vi "MOSES.vi"(7 "Scan List (empty)":string="101:132,201:222", 8 "error in (no error)":errorcluster, 9 "Range (5:Auto)":T3(ring)=enum."Auto", 10 "Resolution (5:Default)":T2(ring)=enum."Default", 11 "VISA resource name":refnum<visa-resource-name>="GPIB0::9::INSTR") -> (0 "error out":errorcluster, 2 "Output Array":dbl[](array[numeric]) format="%.2f", 3 "VISA resource name out":refnum<visa-resource-name>)   [LabVIEW 2013]
doc: "This VI allows you to take simple voltage measurements from the instrument."
uses:
  Instance           7 13Saved   MOSES .vi
  Instance           2 13Saved   MOSES .vi
  Instance          24 13Saved   MOSES .vi
  Instance          83 13Saved   MOSES .vi
  Instance          81 13Saved   MOSES .vi
  Instance          79 13Saved   MOSES .vi
  Instance          77 13Saved   MOSES .vi
  Instance          75 13Saved   MOSES .vi
  Instance          71 13Saved   MOSES .vi
  Instance          69 13Saved   MOSES .vi
  Instance          67 13Saved   MOSES .vi
  Instance          65 13Saved   MOSES .vi
  Instance          63 13Saved   MOSES .vi
  Instance          61 13Saved   MOSES .vi
  Instance          59 13Saved   MOSES .vi
  Instance          57 13Saved   MOSES .vi
  Instance          55 13Saved   MOSES .vi
  Instance          53 13Saved   MOSES .vi
  Instance          51 13Saved   MOSES .vi
  Instance          49 13Saved   MOSES .vi
  Instance          47 13Saved   MOSES .vi
  Instance          42 13Saved   MOSES .vi
  Instance          40 13Saved   MOSES .vi
  Instance          38 13Saved   MOSES .vi
  Instance          36 13Saved   MOSES .vi
  Instance          34 13Saved   MOSES .vi
  Instance          32 13Saved   MOSES .vi
  Instance          30 13Saved   MOSES .vi
  Instance          28 13Saved   MOSES .vi
  Instance          26 13Saved   MOSES .vi
  Instance          22 13Saved   MOSES .vi
  Instance          20 13Saved   MOSES .vi
  Instance          18 13Saved   MOSES .vi
  Instance          16 13Saved   MOSES .vi
  Instance          14 13Saved   MOSES .vi
  Instance          12 13Saved   MOSES .vi
  Instance          10 13Saved   MOSES .vi
  Instance           8 13Saved   MOSES .vi
  <vilib>/express/express shared/transition.llb/Dynamic To Waveform Array.vi
  <vilib>/express/express shared/transition.llb/Waveform Array To Dynamic.vi
  <vilib>/express/express arith-compare/Formula/Block/exnFormulaBlock how many pts in the wave.vi
  <vilib>/express/express shared/ex_Modify Signal Name.vi
  <vilib>/express/express arith-compare/Formula/XNode/ExpressFormulaBlockNode.xnode
panel:
  in  "?":bool
  in  "?":T1(tab)
  out "TEC L -y":dbl
  out "Battery":dbl
  out "Boolean 10":bool
  out "Boolean 11":bool
  out "Boolean 12":bool
  out "Mains from IS":dbl
  out "Boolean 13":bool
  out "Boolean 14":bool
  out "Boolean 15":bool
  out "12d+, MTR2812D Out":dbl
  out "Boolean 16":bool
  out "Boolean 17":bool
  out "5s, MGA2805S Out":dbl
  out "Boolean 26":bool
  out "Boolean 27":bool
  out "IS Out":dbl
  out "Boolean 20":bool
  out "Boolean 21":bool
  out "Boolean 22":bool
  out "12d+ MTR2812D Out":dbl
  out "Boolean 23":bool
  out "Boolean 24":bool
  out "Boolean 25":bool
  out "5s MGA2805S Out":dbl
  out "Boolean 29":bool
  out "Boolean 30":bool
  out "Boolean 31":bool
  out "Power Supply Filter Input":dbl
  out "Boolean 67":bool
  out "Boolean 68":bool
  out "Boolean 90":bool
  out "Boolean 7":bool
  out "Boolean 8":bool
  out "TEC L +y":dbl
  out "Boolean 6":bool
  out "Boolean 5":bool
  out "TEC L 0y":dbl
  out "Boolean 9":bool
  out "Boolean 18":bool
  out "TEC R +y":dbl
  out "Boolean 19":bool
  out "Boolean 45":bool
  out "TEC R -y":dbl
  out "Boolean 46":bool
  out "Boolean 75":bool
  out "TEC R 0y":dbl
  out "Boolean 76":bool
  out "Boolean 89":bool
  out "Thermal 5V power":dbl
  out "Shutter 28V power":dbl
  out "H-alpha filter":dbl
  out "H-alpha camera":dbl
  out "ROE power supply input":dbl
  out "Premod filter positive 12V input":dbl
  out "Premod filter 5V input":dbl
  out "Shutter 28V power":dbl
  out "H-alpha filter":dbl
  out "ROE power supply input":dbl
  out "Boolean 41":bool
  out "Boolean 42":bool
  out "Res +y":dbl
  out "Res -y":dbl
  out "Res Back":dbl
  out "Boolean 43":bool
  out "Boolean 44":bool
  out "Boolean 47":bool
  out "Boolean 48":bool
  out "Boolean 49":bool
  out "Boolean 50":bool
  out "CF +y":dbl
  out "CF -y":dbl
  out "CF 0y":dbl
  out "Boolean 51":bool
  out "Boolean 52":bool
  out "Boolean 53":bool
  out "Boolean 54":bool
  out "BP +y":dbl
  out "BP -y":dbl
  out "BP 0y":dbl
  out "Boolean 55":bool
  out "Boolean 56":bool
  out "Boolean 57":bool
  out "Boolean 58":bool
  out "Boolean 59":bool
  out "Boolean 60":bool
  out "Boolean 40":bool
  out "PCU Res":dbl
  out "Boolean 83":bool
  out "Boolean 84":bool
  out "ICU":dbl
  out "Boolean 85":bool
  out "Boolean 86":bool
  out "PCU Box":dbl
  out "Boolean 87":bool
  out "Boolean 88":bool
  out "Boolean 32":bool
  out "Boolean 33":bool
  out "Boolean 34":bool
  out "TEC +y":dbl
  out "TEC -y":dbl
  out "TEC 0y":dbl
  out "Boolean 35":bool
  out "Boolean 36":bool
  out "Boolean 37":bool
  out "Boolean 38":bool
  out "Boolean 39":bool
  out "Comp Res":dbl
  out "Boolean 61":bool
  out "Boolean 62":bool
  out "Vortec x86 CPU":dbl
  out "Boolean 63":bool
  out "Boolean 64":bool
  out "Mainboard":dbl
  out "Boolean 65":bool
  out "Boolean 66":bool
  out "Virtex 5 FPGA":dbl
  out "Boolean 69":bool
  out "Boolean 70":bool
  out "RPA":dbl
  out "Boolean 71":bool
  out "Boolean 72":bool
  out "TC Res.":dbl
  out "Boolean 73":bool
  out "Boolean 74":bool
  out "T CONT b -y":dbl
  out "Boolean 77":bool
  out "Boolean 78":bool
  out "12S":dbl
  out "Boolean 79":bool
  out "Boolean 80":bool
  out "12D":dbl
  out "Boolean 81":bool
  out "Boolean 82":bool
  out "0 Order TECs":dbl[][](graph)
  out "-1 Order TECs":dbl[][](graph)
  out "+1 Order TECs":dbl[][](graph)
  out "I5s":dbl[](graph)
  out "I12d+":dbl[](graph)
  out "Iout":dbl[](graph)
  out "Power Supply Filter Input":dbl[](graph)
  out "TEC Currents":dbl[][](graph)
  out "Back Plates":dbl[][](graph)
  out "Cold Fingers":dbl[][](graph)
  out "CONT":dbl[][](graph)
  out "PCU":dbl[][](graph)
  out "COMP":dbl[][](graph)
  out "Reservoir":dbl[][](graph)
  out "ROE":dbl[](graph)
  out "PSU":dbl[](graph)
  in  "C":dbl
  in  "B":dbl
  in  "A":dbl
  in  "stop 2":bool
  # "System"
  # "System"
  # "Voltage"
  # "Current"
  # "C"
  # "V"
  # "A"
  # "Temperatures of \n+1 Order CCD\nThermal Reservoir, Cold Finger, and Back Plate"
  # "C"
  # "A"
  # "V"
  # "C"
  # "A"
  # "V"
  # "Temperatures of \n0 Order CCD\nCold Finger and Back Plate"
  # "C"
  # "V"
  # "mA"
  # "C"
  # "Thermo Electric Coolers (TEC)"
  # "CCD"
  # "Voltage on L or R side of TEC"
  # "Current"
  # "C"
  # "Temperatures of \n-1 Order CCD\nThermal Reservoir, Cold Finger, and Back Plate"
  # "V"
  # "C"
  # "+1 Order"
  # "A"
  # "V"
  # "C"
  # "Temperature of\nBack of Thermal Reservoir"
  # "C"
  # "V"
  # "0 Order"
  # "A"
  # "Computer"
  # "V"
  # "C"
  # "C"
  # "C"
  # "V"
  # "-1 Order"
  # "A"
  # "C"
  # "C"
  # "C"
  # "V"
  # "Sub-Systems"
  # "C"
  # "C"
  # "Current"
  # "Voltage"
  # "C"
  # "C"
  # "mA"
  # "V"
  # "C"
  # "C"
  # "V"
  # "mA"
  # "V"
  # "A"
  # "V"
  # "A"
  # "V"
  # "A"
  # "Please add graphs and values that you would like to see in the text box below."
  # "Flight Screen:\n-TECs\n-\n-"
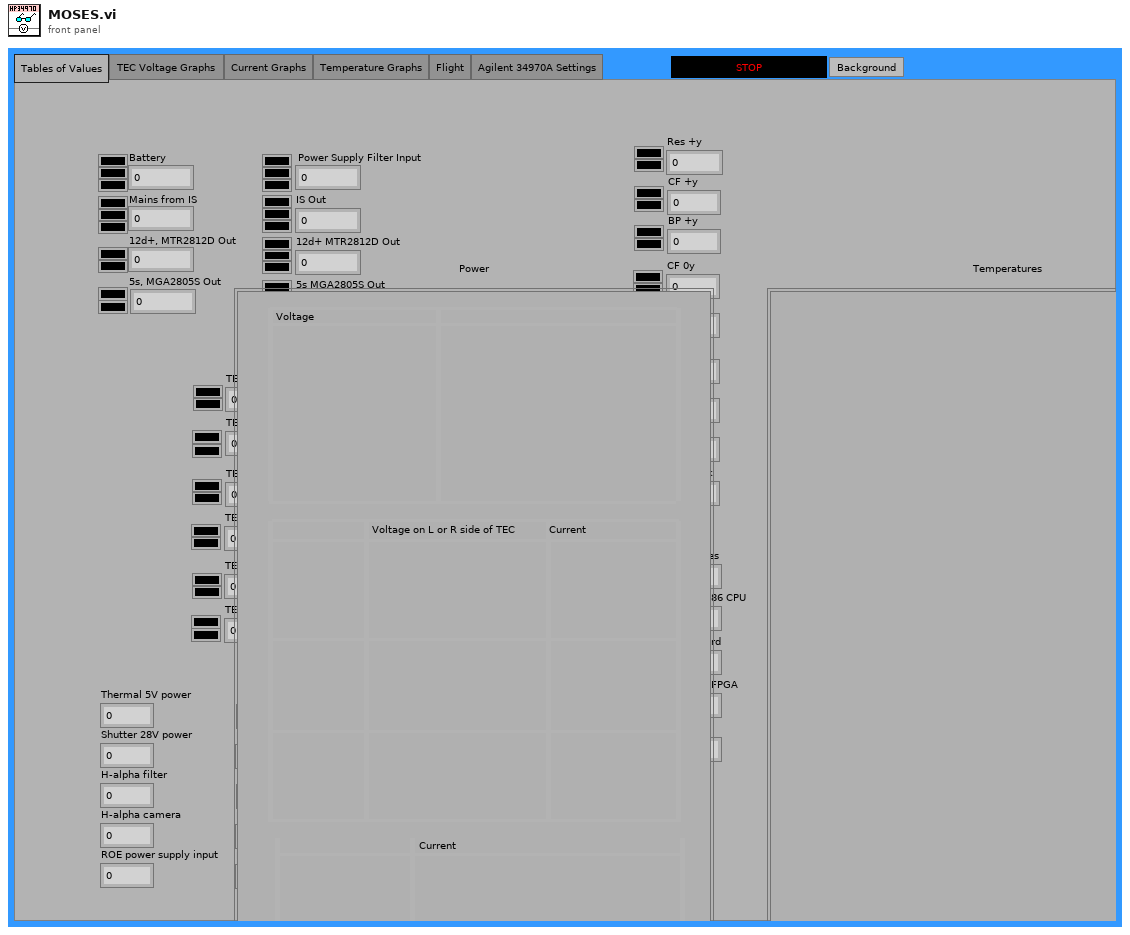
[diagram p1: front panel]
types:
  T1 = enum32{"Tables of Values", "TEC Voltage Graphs ", "Current Graphs", "Temperature Graphs", "Flight", "Agilent 34970A Settings"}
  T2 = enum16{"4 1/2", "5 1/2", "6 1/2", "Least", "Highest", "Default"}
  T3 = enum16{"100 mV", "1 V", "10 V", "100 V", "300 V", "Auto", "Minimum", "Maximum"}
  T4 = cluster{"Output Number Array[0]":dbl, "Output Number Array[1]":dbl, "Output Number Array[2]":dbl, "Output Number Array[3]":dbl, "Output Number Array[4]":dbl, "Output Number Array[5]":dbl, "Output Number Array[6]":dbl, "Output Number Array[7]":dbl, "Output Number Array[8]":dbl, "Output Number Array[9]":dbl, "Output Number Array[10]":dbl, "Output Number Array[11]":dbl, "Output Number Array[12]":dbl, "Output Number Array[13]":dbl, "Output Number Array[14]":dbl, "Output Number Array[15]":dbl, "Output Number Array[16]":dbl, "Output Number Array[17]":dbl, "Output Number Array[18]":dbl, "Output Number Array[19]":dbl, "Output Number Array[20]":dbl, "Output Number Array[21]":dbl, "Output Number Array[22]":dbl, "Output Number Array[23]":dbl, "Output Number Array[24]":dbl, "Output Number Array[25]":dbl, "Output Number Array[26]":dbl, "Output Number Array[27]":dbl, "Output Number Array[28]":dbl, "Output Number Array[29]":dbl, "Output Number Array[30]":dbl, "Output Number Array[31]":dbl, "Output Number Array[32]":dbl, "Output Number Array[33]":dbl, "Output Number Array[34]":dbl, "Output Number Array[35]":dbl, "Output Number Array[36]":dbl, "Output Number Array[37]":dbl, "Output Number Array[38]":dbl, "Output Number Array[39]":dbl, "Output Number Array[40]":dbl, "Output Number Array[41]":dbl, "Output Number Array[42]":dbl, "Output Number Array[43]":dbl, "Output Number Array[44]":dbl, "Output Number Array[45]":dbl, "Output Number Array[46]":dbl, "Output Number Array[47]":dbl, "Output Number Array[48]":dbl, "Output Number Array[49]":dbl, "Output Number Array[50]":dbl, "Output Number Array[51]":dbl, "Output Number Array[52]":dbl, "Output Number Array[53]":dbl, "Output Number Array[54]":dbl, "Output Number Array[55]":dbl, "Output Number Array[56]":dbl, "Output Number Array[57]":dbl, "Output Number Array[58]":dbl, "Output Number Array[59]":dbl, "Output Number Array[60]":dbl, "Output Number Array[61]":dbl, "Output Number Array[62]":dbl, "Output Number Array[63]":dbl, "Output Number Array[64]":dbl, "Output Number Array[65]":dbl, "Output Number Array[66]":dbl, "Output Number Array[67]":dbl, "Output Number Array[68]":dbl, "Output Number Array[69]":dbl}
  T5 = cluster{"V5s, MGA2805S output voltage":dbl, "T5V, Thermal 5V power voltage":dbl, "S28V, Shutter 28V power voltage":dbl, "HAFV, H-alpha filter voltage":dbl, "HACV, H-alpha camera voltage":dbl, "If_in, Power supply filter input current":dbl, "Ipf12+, Premod filter positive 12V input current":dbl, "I_pf5, Premod filter 5V input current":dbl, "S28I, Shutter 28V power current":dbl, "HAFI, H-alpha filter current":dbl, "ROE_PSV, ROE power supply input voltage":dbl, "ROE_PSI, ROE power supply input current":dbl, "T_ROE, ROE Temp.":dbl, "T_PSU, PSU Temp.":dbl}
diagram:
  # "This goes to MOSES background."
  n1 = while {
    shift-right: [w645] -> _
    shift-left: _ -> [w646]
    shift-right: [w1] -> _
    shift-left: _ -> [w637]
    shift-right: [w635] -> _
    shift-left: _ -> [w636]
    shift-right: [w2] -> _
    shift-left: _ -> [w620]
    shift-right: [w3] -> _
    shift-left: _ -> [w618]
    shift-right: [w4] -> _
    shift-left: _ -> [w597]
    shift-right: [w5] -> _
    shift-left: _ -> [w593]
    shift-right: [w6] -> _
    shift-left: _ -> [w182]
    shift-right: [w7] -> _
    shift-left: _ -> [w580]
    shift-right: [w8] -> _
    shift-left: _ -> [w563]
    shift-right: [w9] -> _
    shift-left: _ -> [w532]
    shift-right: [w10] -> _
    shift-left: _ -> [w511]
    shift-right: [w505] -> _
    shift-left: _ -> [w506]
    shift-right: [w463] -> _
    shift-left: _ -> [w462]
    shift-right: [w461] -> _
    shift-left: _ -> [w460]
    shift-right: [w457] -> _
    shift-left: _ -> [w458]
    shift-right: [w456] -> _
    shift-left: _ -> [w455]
    shift-right: [w454] -> _
    shift-left: _ -> [w453]
    shift-right: [w452] -> _
    shift-left: _ -> [w451]
    shift-right: [w450] -> _
    shift-left: _ -> [w449]
    shift-right: [w448] -> _
    shift-left: _ -> [w183]
    shift-right: [w447] -> _
    shift-left: _ -> [w446]
    shift-right: [w445] -> _
    shift-left: _ -> [w444]
    shift-right: [w443] -> _
    shift-left: _ -> [w442]
    shift-right: [w63] -> _
    shift-left: _ -> [w176]
    shift-right: [w434] -> _
    shift-left: _ -> [w433]
    shift-right: [w89] -> _
    shift-left: _ -> [w435]
    shift-right: [w432] -> _
    shift-left: _ -> [w431]
    shift-right: [w430] -> _
    shift-left: _ -> [w429]
    shift-right: [w11] -> _
    shift-left: _ -> [w368]
    shift-right: [w366] -> _
    shift-left: _ -> [w367]
    shift-right: [w365] -> _
    shift-left: _ -> [w364]
    shift-right: [w363] -> _
    shift-left: _ -> [w362]
    shift-right: [w360] -> _
    shift-left: _ -> [w361]
    shift-right: [w356] -> _
    shift-left: _ -> [w357]
    shift-right: [w359] -> _
    shift-left: _ -> [w358]
    shift-right: [w12] -> _
    shift-left: _ -> [w316]
    shift-right: [w314] -> _
    shift-left: _ -> [w313]
    shift-right: [w312] -> _
    shift-left: _ -> [w311]
    shift-right: [w309] -> _
    shift-left: _ -> [w310]
    shift-right: [w308] -> _
    shift-left: _ -> [w307]
    shift-right: [w273] -> _
    shift-left: _ -> [w274]
    shift-right: [w272] -> _
    shift-left: _ -> [w271]
    shift-right: [w269] -> _
    shift-left: _ -> [w270]
    shift-right: [w13] -> _
    shift-left: _ -> [w275]
    stop <- "stop 2" stop-if-true
    w75 = 0.05 ("y")
    w76 = 4.0 ("y")
    w81 = 2.5 ("y")
    w119 = 2.5 ("y")
    w123 = 2.5 ("y")
    w127 = 2.5 ("y")
    w130 = 2.5 ("y")
    (unwired) 37482.0 ("double precision float")
    (unwired) 9360000.0 ("double precision float")
    (unwired) 9.3e-08 ("double precision float")
    (unwired) 0.000236053 ("double precision float")
    (unwired) 9.3e-08 ("double precision float")
    (unwired) 0.000236053 ("double precision float")
    (unwired) 0.001285847 ("double precision float")
    (unwired) 0.001285847 ("double precision float")
    w69 = 150.0 ("y")
    w73 = 300.0 ("y")
    w104 = 2.5 ("y")
    w22 = 0.03 ("y")
    w109 = 3.0 ("y")
    w29 = 0.01 ("y")
    w639 = 2.5 ("y")
    w641 = 2.5 ("y")
    # "File saves to data.txt on the desktop."
    # "These four need real equations and alarm limits."
    # "For highest resolution\nmeasurements, \nchange VISA timeout"
    n2 = Append True/False String(1:FALSE ("selector"), 2:"DC? ", 3:"AC? ", 4:"MEAS:VOLT:") -> (0:w653:string)
    n3 = Pick Line(string ("")=w653, multi-line string=".1,\n1,\n10,\n100,\n300,\nAUTO\nMIN,\nMAX,", line index="Range (5:Auto)") -> (output string=w650:string)
    n4 = case shown="Default" "Range (5:Auto)" {
      selector: "Range (5:Auto)" -> [_ w1550]
      tunnel: [w1544 w1547] -> w649
      tunnel: w650 -> [w1544 w1546]
      tunnel: "Resolution (5:Default)" -> [_ w1548]
      frame "Auto" {
        # "Autorange"
      }
      frame Default {
        # "Not Autorange"
        n5 = Index Array(array=dbl[] [0.1, 1.0, 10.0, 100.0, 300.0, 0.0, 0.1, 300.0], index=w1550) -> (element=w1545:dbl)
        n6 = case shown="Default" w1548 {
          selector: w1548 -> [w1557 _ _ _]
          tunnel: [w1551 w1561 w1564 w1565] -> w1547
          tunnel: w1546 -> [w1554 w1560 w1562 w1566]
          tunnel: w1545 -> [w1556 _ _ _]
          frame Default {
            # "4.5, 5.5, or 6.5 Digits *"
            n7 = Index Array(array=dbl[] [0.0001, 3e-06, 1e-06], index=w1557) -> (element=w1555:dbl)
            n8 = Multiply(x=w1555, y=w1556) -> (x*y=w1553:dbl)
            n9 = Format Into String(format string="%.; %e", initial string=w1554, w1553) -> (resulting string=w1551:string)  [unwired: 1 in, 1 out]
          }
          frame "Least" {
            # "Least resolution"
            n10 = Concatenate Strings(w1560, " MAX" ("string")) -> (w1561:string)
          }
          frame "Highest" {
            # "Highest range"
            n11 = Concatenate Strings(w1562, " MIN" ("string")) -> (w1564:string)
          }
          frame "Default" {
            # "Default range"
            n12 = Concatenate Strings(w1566, " DEF" ("string")) -> (w1565:string)
          }
        }
      }
    }
    n13 = call "Convert to Dynamic Data3"() -> ("Dynamic Data Type"=w577:dynamicdata)  [unwired: 4 in]
    n14 = xnode "Voltage - Resistance"("V1"=5000, "28V"=w577, "R1"=28) -> ("Result"=w572:dynamicdata)  [unwired: 1 in, 1 out]
    n15 = Concatenate Strings(w649, ", (@", "Scan List (empty)", ")") -> (w660:string)
    n16 = VISA Write(VISA resource name="VISA resource name", write buffer=w660, error in (no error)="error in (no error)") -> (VISA resource name out=w669:refnum<visa-resource-name>, error out=w668:errorcluster)  [unwired: 1 out]
    n17 = xnode "Steinhart-Hart"("X1"=5000, "X2"=5000, "X3"=5000, "X4"=w572) -> ("Result"=w578:dynamicdata)  [unwired: 1 in, 1 out]
    n18 = property class="Instr"(reference=w669, error in=w668, "General Settings:Timeout Value"=u32 320000 ("Tmo Value")) -> (reference out=w666:refnum<visa-resource-name>, error out=w667:errorcluster)
    n19 = call "Convert from Dynamic Data9"("Dynamic Data Type"=w578) -> ()  [unwired: 3 in, 1 out]
    n20 = Get Date/Time String(want seconds? (F)=TRUE) -> (time string=w648:string)  [unwired: 2 in, 1 out]
    n21 = VISA Read(VISA resource name=w666, byte count=u32 4088 ("byte count (0)"), error in (no error)=w667) -> (VISA resource name out=→"VISA resource name out":refnum<visa-resource-name>, read buffer=w661:string, error out=→"error out":errorcluster)  [unwired: 1 out]
    n22 = call <instrlib>:"HP34970A List to Array.vi"("List (empty)"=w661) -> ("Output Number Array"=w181:dbl[])  [unwired: 5 in, 1 out]
    "Output Array" <- w181
    n23 = call "sub_vi.vi"("Array"=w181) -> ("Dynamic Data Type"=w643:dynamicdata)  [unwired: 3 in]
    n24 = call "Write LabVIEW Measurement File2"("Comment"=w648, "Signals"=w643) -> ()  [unwired: 7 in, 3 out]
    n25 = Array To Cluster(array=w181) -> (cluster=w638:T4)
    n26 = Build Array (concatenate)(w646, w181) -> (w645:dbl[][])
    n27 = Unbundle(w638) -> ("Output Number Array[0]"=w134:dbl, "Output Number Array[1]"=w20:dbl, "Output Number Array[2]"=w132:dbl, "Output Number Array[3]"=w126:dbl, "Output Number Array[4]"=w122:dbl, "Output Number Array[5]"=w118:dbl, "Output Number Array[8]"=w140:dbl, "Output Number Array[9]"=w143:dbl, "Output Number Array[10]"=w146:dbl, "Output Number Array[11]"=w98:dbl, "Output Number Array[16]"=w175:dbl, "Output Number Array[17]"=w88:dbl, "Output Number Array[18]"=w174:dbl, "Output Number Array[19]"=w173:dbl, "Output Number Array[22]"=w172:dbl, "Output Number Array[23]"=w171:dbl, "Output Number Array[24]"=w170:dbl, "Output Number Array[29]"=w169:dbl, "Output Number Array[30]"=w168:dbl, "Output Number Array[32]"=w167:dbl, "Output Number Array[33]"=w166:dbl, "Output Number Array[34]"=w165:dbl, "Output Number Array[35]"=w164:dbl, "Output Number Array[36]"=w163:dbl, "Output Number Array[37]"=w162:dbl, "Output Number Array[38]"=w161:dbl, "Output Number Array[39]"=w160:dbl, "Output Number Array[40]"=w159:dbl, "Output Number Array[41]"=w158:dbl, "Output Number Array[42]"=w157:dbl, "Output Number Array[43]"=w156:dbl, "Output Number Array[44]"=w155:dbl, "Output Number Array[45]"=w154:dbl, "Output Number Array[46]"=w147:dbl, "Output Number Array[49]"=w151:dbl, "Output Number Array[50]"=w152:dbl, "Output Number Array[51]"=w150:dbl, "Output Number Array[52]"=w148:dbl, "Output Number Array[53]"=w149:dbl)  [unwired: 31 out]
    "TEC L +y" <- w134
    "TEC L 0y" <- w132
    "TEC R +y" <- w126
    "TEC R -y" <- w122
    "TEC R 0y" <- w118
    "TEC L -y" <- w20
    n28 = xnode "Votage - Current"("X1"=w172) -> ("Result"=w583:dbl)  [unwired: 1 in, 1 out]
    n29 = xnode "V -> T"("a"=0.001285847 ("double precision float"), "b"=0.000236053 ("double precision float"), "c"=9.3e-08 ("double precision float"), "R"=9360000.0 ("double precision float"), "v0"=w169) -> ("Result"=w566:dbl)  [unwired: 1 in, 1 out]
    n30 = xnode "V -> T"("a"=0.001285847 ("double precision float"), "b"=0.000236053 ("double precision float"), "c"=9.3e-08 ("double precision float"), "R"=9360000.0 ("double precision float"), "v0"=w167) -> ("Result"=w551:dbl)  [unwired: 1 in, 1 out]
    n31 = xnode "V -> T"("a"=0.001285847 ("double precision float"), "b"=0.000236053 ("double precision float"), "c"=9.3e-08 ("double precision float"), "R"=1420000.0 ("double precision float"), "v0"=w166) -> ("Result"=w545:dbl)  [unwired: 1 in, 1 out]
    n32 = xnode "V -> T"("a"=0.001285847 ("double precision float"), "b"=0.000236053 ("double precision float"), "c"=9.3e-08 ("double precision float"), "R"=1420000.0 ("double precision float"), "v0"=w162) -> ("Result"=w519:dbl)  [unwired: 1 in, 1 out]
    n33 = xnode "V -> T"("a"=0.001285847 ("double precision float"), "b"=0.000236053 ("double precision float"), "c"=9.3e-08 ("double precision float"), "R"=37482.0 ("double precision float"), "v0"=w149) -> ("Result"=w323:dbl)  [unwired: 1 in, 1 out]
    n34 = xnode "V -> T"("a"=0.001285847 ("double precision float"), "b"=0.000236053 ("double precision float"), "c"=9.3e-08 ("double precision float"), "R"=37482.0 ("double precision float"), "v0"=w152) -> ("Result"=w283:dbl)  [unwired: 1 in, 1 out]
    n35 = xnode "Votage - Current"("X1"=w171) -> ("Result"=w582:dbl)  [unwired: 1 in, 1 out]
    n36 = xnode "Votage - Current"("X1"=w170) -> ("Result"=w581:dbl)  [unwired: 1 in, 1 out]
    n37 = xnode "V -> T"("a"=0.001285847 ("double precision float"), "b"=0.000236053 ("double precision float"), "c"=9.3e-08 ("double precision float"), "R"=1420000.0 ("double precision float"), "v0"=w164) -> ("Result"=w533:dbl)  [unwired: 1 in, 1 out]
    n38 = xnode "V -> T"("a"=0.001285847 ("double precision float"), "b"=0.000236053 ("double precision float"), "c"=9.3e-08 ("double precision float"), "R"=37482.0 ("double precision float"), "v0"=w148) -> ("Result"=w332:dbl)  [unwired: 1 in, 1 out]
    n39 = xnode "V -> T"("a"=0.001285847 ("double precision float"), "b"=0.000236053 ("double precision float"), "c"=9.3e-08 ("double precision float"), "R"=37482.0 ("double precision float"), "v0"=w150) -> ("Result"=w292:dbl)  [unwired: 1 in, 1 out]
    n40 = xnode "V -> T"("a"=0.001285847 ("double precision float"), "b"=0.000236053 ("double precision float"), "c"=9.3e-08 ("double precision float"), "R"=9360000.0 ("double precision float"), "v0"=w168) -> ("Result"=w557:dbl)  [unwired: 1 in, 1 out]
    n41 = xnode "V -> T"("a"=0.001285847 ("double precision float"), "b"=0.000236053 ("double precision float"), "c"=9.3e-08 ("double precision float"), "R"=1420000.0 ("double precision float"), "v0"=w163) -> ("Result"=w525:dbl)  [unwired: 1 in, 1 out]
    n42 = xnode "V -> T"("a"=0.001285847 ("double precision float"), "b"=0.000236053 ("double precision float"), "c"=9.3e-08 ("double precision float"), "R"=1420000.0 ("double precision float"), "v0"=w161) -> ("Result"=w513:dbl)  [unwired: 1 in, 1 out]
    n43 = xnode "V -> T"("a"=0.001285847 ("double precision float"), "b"=0.000236053 ("double precision float"), "c"=9.3e-08 ("double precision float"), "R"=37482.0 ("double precision float"), "v0"=w158) -> ("Result"=w404:dbl)  [unwired: 1 in, 1 out]
    n44 = xnode "V -> T"("a"=0.001285847 ("double precision float"), "b"=0.000236053 ("double precision float"), "c"=9.3e-08 ("double precision float"), "R"=37482.0 ("double precision float"), "v0"=w157) -> ("Result"=w396:dbl)  [unwired: 1 in, 1 out]
    n45 = xnode "V -> T"("a"=0.001285847 ("double precision float"), "b"=0.000236053 ("double precision float"), "c"=9.3e-08 ("double precision float"), "R"=37482.0 ("double precision float"), "v0"=w154) -> ("Result"=w350:dbl)  [unwired: 1 in, 1 out]
    n46 = xnode "V -> T"("a"=0.001285847 ("double precision float"), "b"=0.000236053 ("double precision float"), "c"=9.3e-08 ("double precision float"), "R"=37482.0 ("double precision float"), "v0"=w151) -> ("Result"=w301:dbl)  [unwired: 1 in, 1 out]
    n47 = xnode "V -> T"("a"=0.001285847 ("double precision float"), "b"=0.000236053 ("double precision float"), "c"=9.3e-08 ("double precision float"), "R"=1420000.0 ("double precision float"), "v0"=w165) -> ("Result"=w539:dbl)  [unwired: 1 in, 1 out]
    n48 = xnode "V -> T"("a"=0.001285847 ("double precision float"), "b"=0.000236053 ("double precision float"), "c"=9.3e-08 ("double precision float"), "R"=291400.0 ("double precision float"), "v0"=w160) -> ("Result"=w422:dbl)  [unwired: 1 in, 1 out]
    n49 = xnode "V -> T"("a"=0.001285847 ("double precision float"), "b"=0.000236053 ("double precision float"), "c"=9.3e-08 ("double precision float"), "R"=37482.0 ("double precision float"), "v0"=w155) -> ("Result"=w378:dbl)  [unwired: 1 in, 1 out]
    n50 = xnode "V -> T"("a"=0.001285847 ("double precision float"), "b"=0.000236053 ("double precision float"), "c"=9.3e-08 ("double precision float"), "R"=37482.0 ("double precision float"), "v0"=w159) -> ("Result"=w413:dbl)  [unwired: 1 in, 1 out]
    n51 = xnode "V -> T"("a"=0.001285847 ("double precision float"), "b"=0.000236053 ("double precision float"), "c"=9.3e-08 ("double precision float"), "R"=37482.0 ("double precision float"), "v0"=w156) -> ("Result"=w387:dbl)  [unwired: 1 in, 1 out]
    n52 = xnode "V -> T"("a"=0.001285847 ("double precision float"), "b"=0.000236053 ("double precision float"), "c"=9.3e-08 ("double precision float"), "R"=37482.0 ("double precision float"), "v0"=w147) -> ("Result"=w341:dbl)  [unwired: 1 in, 1 out]
    n53 = xnode "Votage - Current 6"("X1"=w174) -> ("Result"=w594:dbl)  [unwired: 1 in, 1 out]
    n54 = xnode "Votage - Current"("X1"=w88) -> ("Result"=w90:dbl)  [unwired: 1 in, 1 out]
    n55 = xnode "Votage - Current 7"("X1"=w175) -> ("Result"=w598:dbl)  [unwired: 1 in, 1 out]
    n56 = xnode "Votage - Current 5"("X1"=w173) -> ("Result"=w589:dbl)  [unwired: 1 in, 1 out]
    n57 = xnode "Votage - Voltage 3"("X1"=w143) -> ("Result"=w142:dbl)  [unwired: 1 in, 1 out]
    n58 = xnode "Votage - Voltage 4"("X1"=w146) -> ("Result"=w145:dbl)  [unwired: 1 in, 1 out]
    n59 = xnode "Votage - Voltage 2"("X1"=w140) -> ("Result"=w141:dbl)  [unwired: 1 in, 1 out]
    n60 = xnode "Votage - Voltage"("X1"=w98) -> ("Result"=w99:dbl)  [unwired: 1 in, 1 out]
    n61 = call "Convert from Dynamic Data11"("Dynamic Data Type"=w557) -> ("Scalar"=w14:dbl)  [unwired: 3 in]
    "Res -y" <- w14
    n62 = call "Convert from Dynamic Data32"("Dynamic Data Type"=w292) -> ("Scalar"=w278:dbl)  [unwired: 3 in]
    "ICU" <- w278
    n63 = call "Convert from Dynamic Data33"("Dynamic Data Type"=w283) -> ("Scalar"=w277:dbl)  [unwired: 3 in]
    "PCU Box" <- w277
    n64 = call "Convert from Dynamic Data7"("Dynamic Data Type"=w582) -> ("Scalar"=w48:dbl)  [unwired: 3 in]
    "TEC -y" <- w48
    n65 = call "Convert from Dynamic Data8"("Dynamic Data Type"=w581) -> ("Scalar"=w37:dbl)  [unwired: 3 in]
    "TEC 0y" <- w37
    n66 = call "Convert from Dynamic Data10"("Dynamic Data Type"=w566) -> ("Scalar"=w565:dbl)  [unwired: 3 in]
    "Res +y" <- w565
    n67 = call "Convert from Dynamic Data13"("Dynamic Data Type"=w551) -> ("Scalar"=w15:dbl)  [unwired: 3 in]
    "Res Back" <- w15
    n68 = call "Convert from Dynamic Data14"("Dynamic Data Type"=w545) -> ("Scalar"=w531:dbl)  [unwired: 3 in]
    "CF +y" <- w531
    n69 = call "Convert from Dynamic Data29"("Dynamic Data Type"=w332) -> ("Scalar"=w318:dbl)  [unwired: 3 in]
    "12S" <- w318
    n70 = call "Convert from Dynamic Data30"("Dynamic Data Type"=w323) -> ("Scalar"=w317:dbl)  [unwired: 3 in]
    "12D" <- w317
    n71 = call "Convert from Dynamic Data6"("Dynamic Data Type"=w583) -> ("Scalar"=w64:dbl)  [unwired: 3 in]
    "TEC +y" <- w64
    n72 = call "Convert from Dynamic Data15"("Dynamic Data Type"=w539) -> ("Scalar"=w18:dbl)  [unwired: 3 in]
    "CF -y" <- w18
    n73 = call "Convert from Dynamic Data16"("Dynamic Data Type"=w533) -> ("Scalar"=w19:dbl)  [unwired: 3 in]
    "CF 0y" <- w19
    n74 = call "Convert from Dynamic Data17"("Dynamic Data Type"=w525) -> ("Scalar"=w510:dbl)  [unwired: 3 in]
    "BP +y" <- w510
    n75 = call "Convert from Dynamic Data18"("Dynamic Data Type"=w519) -> ("Scalar"=w16:dbl)  [unwired: 3 in]
    "BP -y" <- w16
    n76 = call "Convert from Dynamic Data19"("Dynamic Data Type"=w513) -> ("Scalar"=w17:dbl)  [unwired: 3 in]
    "BP 0y" <- w17
    n77 = call "Convert from Dynamic Data28"("Dynamic Data Type"=w341) -> ("Scalar"=w153:dbl)  [unwired: 3 in]
    "T CONT b -y" <- w153
    n78 = call "Convert from Dynamic Data31"("Dynamic Data Type"=w301) -> ("Scalar"=w279:dbl)  [unwired: 3 in]
    "PCU Res" <- w279
    n79 = call "Convert from Dynamic Data5"("Dynamic Data Type"=w589) -> ("Scalar"=w70:dbl)  [unwired: 3 in]
    "5s MGA2805S Out" <- w70
    n80 = call "Convert from Dynamic Data20"("Dynamic Data Type"=w422) -> ("Scalar"=w374:dbl)  [unwired: 3 in]
    "Comp Res" <- w374
    n81 = call "Convert from Dynamic Data26"("Dynamic Data Type"=w350) -> ("Scalar"=w319:dbl)  [unwired: 3 in]
    "TC Res." <- w319
    n82 = call "Convert from Dynamic Data3"("Dynamic Data Type"=w594) -> ("Scalar"=w105:dbl)  [unwired: 3 in]
    "12d+ MTR2812D Out" <- w105
    n83 = Less?(x=w105, y=w104) -> (x < y?=w21:bool)
    n84 = Absolute Value(x=w105) -> (abs(x)=w23:dbl)
    n85 = call "Convert from Dynamic Data21"("Dynamic Data Type"=w413) -> ("Scalar"=w373:dbl)  [unwired: 3 in]
    "Vortec x86 CPU" <- w373
    n86 = call "Convert from Dynamic Data22"("Dynamic Data Type"=w404) -> ("Scalar"=w372:dbl)  [unwired: 3 in]
    "Mainboard" <- w372
    n87 = call "Convert from Dynamic Data23"("Dynamic Data Type"=w396) -> ("Scalar"=w100:dbl)  [unwired: 3 in]
    n88 = call "Convert from Dynamic Data24"("Dynamic Data Type"=w387) -> ("Scalar"=w371:dbl)  [unwired: 3 in]
    "Virtex 5 FPGA" <- w371
    n89 = call "Convert from Dynamic Data25"("Dynamic Data Type"=w378) -> ("Scalar"=w370:dbl)  [unwired: 3 in]
    "RPA" <- w370
    n90 = call "Convert from Dynamic Data2"("Dynamic Data Type"=w598) -> ("Scalar"=w110:dbl)  [unwired: 3 in]
    "IS Out" <- w110
    n91 = Absolute Value(x=w110) -> (abs(x)=w30:dbl)
    n92 = Less?(x=w110, y=w109) -> (x < y?=w26:bool)
    n93 = Less?(x=w20, y=w641) -> (x < y?=→"Boolean 6":bool)
    n94 = Greater?(x=w70, y=w73) -> (0:w591:bool)
    n95 = Greater?(x=w64, y=2.85) -> (0:→"Boolean 32":bool)
    n96 = Greater?(x=w30, y=w29) -> (0:w27:bool)
    n97 = Greater?(x=w23, y=w22) -> (0:w24:bool)
    n98 = Less?(x=w14, y=-65.0) -> (x < y?=w559:bool)
    n99 = Less?(x=w278, y=0.0) -> (x < y?=w294:bool)
    n100 = Less?(x=w277, y=15.0) -> (x < y?=w285:bool)
    n101 = Less?(x=w565, y=-65.0) -> (x < y?=w568:bool)
    n102 = Less?(x=w15, y=-65.0) -> (x < y?=w553:bool)
    n103 = Less?(x=w531, y=-31.0) -> (x < y?=w547:bool)
    n104 = Less?(x=w318, y=15.0) -> (x < y?=w334:bool)
    n105 = Less?(x=w317, y=15.0) -> (x < y?=w325:bool)
    n106 = Less?(x=w18, y=-31.0) -> (x < y?=w541:bool)
    n107 = Less?(x=w19, y=-31.0) -> (x < y?=w535:bool)
    n108 = Less?(x=w510, y=-55.0) -> (x < y?=w527:bool)
    n109 = Less?(x=w16, y=-55.0) -> (x < y?=w521:bool)
    n110 = Less?(x=w17, y=-55.0) -> (x < y?=w515:bool)
    n111 = Less?(x=w153, y=15.0) -> (x < y?=w343:bool)
    n112 = Less?(x=w279, y=15.0) -> (x < y?=w303:bool)
    n113 = Greater?(x=w48, y=2.75) -> (0:→"Boolean 35":bool)
    n114 = Less?(x=w374, y=0.0) -> (x < y?=w424:bool)
    n115 = Less?(x=w319, y=15.0) -> (x < y?=w352:bool)
    n116 = Greater?(x=w37, y=2.75) -> (0:→"Boolean 38":bool)
    n117 = Less?(x=w373, y=6.0) -> (x < y?=w415:bool)
    n118 = Less?(x=w372, y=6.0) -> (x < y?=w406:bool)
    n119 = Less?(x=w100, y=10.8) -> (x < y?=w397:bool)
    n120 = Less?(x=w371, y=6.0) -> (x < y?=w389:bool)
    n121 = Less?(x=w370, y=6.0) -> (x < y?=w380:bool)
    n122 = call "Convert from Dynamic Data12"("Dynamic Data Type"=w90) -> ("Scalar"=w77:dbl)  [unwired: 3 in]
    "Power Supply Filter Input" <- w77
    n123 = call "Convert from Dynamic Data36"("Dynamic Data Type"=w142) -> ("Scalar"=w114:dbl)  [unwired: 3 in]
    "Mains from IS" <- w114
    n124 = call "Convert from Dynamic Data34"("Dynamic Data Type"=w145) -> ("Scalar"=w112:dbl)  [unwired: 3 in]
    "12d+, MTR2812D Out" <- w112
    n125 = call "Convert from Dynamic Data37"("Dynamic Data Type"=w141) -> ("Scalar"=w139:dbl)  [unwired: 3 in]
    "Battery" <- w139
    n126 = call "Convert to Dynamic Data2"("Array"=w181) -> ("Dynamic Data Type"=w632:dynamicdata)  [unwired: 3 in]
    n127 = And(x=w26, y=w27) -> (x .and. y?=w28:bool)
    "Boolean 20" <- w28
    n128 = And(x=w21, y=w24) -> (x .and. y?=w25:bool)
    "Boolean 23" <- w25
    n129 = Absolute Value(x=w139) -> (abs(x)=w625:dbl)
    n130 = Absolute Value(x=w114) -> (abs(x)=w612:dbl)
    n131 = Greater?(x=w77, y=w76) -> (0:w79:bool)
    n132 = Less?(x=w112, y=10.8) -> (x < y?=w600:bool)
    n133 = Less?(x=w77, y=w75) -> (x < y?=w80:bool)
    n134 = Greater?(x=w14, y=-60.0) -> (0:w560:bool)
    n135 = Greater?(x=w278, y=30.0) -> (0:w295:bool)
    n136 = Greater?(x=w277, y=40.0) -> (0:w286:bool)
    n137 = Greater?(x=w565, y=-60.0) -> (0:w569:bool)
    n138 = Greater?(x=w15, y=-60.0) -> (0:w554:bool)
    n139 = Greater?(x=w531, y=-30.0) -> (0:w548:bool)
    n140 = Greater?(x=w318, y=50.0) -> (0:w335:bool)
    n141 = Greater?(x=w317, y=50.0) -> (0:w326:bool)
    n142 = Greater?(x=w18, y=-30.0) -> (0:w542:bool)
    n143 = Greater?(x=w19, y=-30.0) -> (0:w536:bool)
    n144 = Greater?(x=w510, y=-35.0) -> (0:w528:bool)
    n145 = Greater?(x=w16, y=-35.0) -> (0:w522:bool)
    n146 = Greater?(x=w17, y=-35.0) -> (0:w516:bool)
    n147 = Greater?(x=w153, y=60.0) -> (0:w344:bool)
    n148 = Greater?(x=w279, y=40.0) -> (0:w304:bool)
    n149 = Greater?(x=w374, y=30.0) -> (0:w425:bool)
    n150 = Greater?(x=w319, y=50.0) -> (0:w353:bool)
    n151 = Greater?(x=w373, y=40.0) -> (0:w416:bool)
    n152 = Greater?(x=w372, y=40.0) -> (0:w407:bool)
    n153 = Greater?(x=w100, y=13.2) -> (0:w398:bool)
    n154 = Greater?(x=w371, y=40.0) -> (0:w390:bool)
    n155 = Greater?(x=w370, y=40.0) -> (0:w381:bool)
    n156 = call "Convert from Dynamic Data4"("Dynamic Data Type"=w99) -> ("Scalar"=w91:dbl)  [unwired: 3 in]
    "5s, MGA2805S Out" <- w91
    n157 = Greater?(x=w134, y=w639) -> (0:→"Boolean 8":bool)
    n158 = xnode "Voltage - Resistance"("X1"=5000, "X2"=w632, "X3"=28) -> ()  [unwired: 1 in, 2 out]
    n159 = Greater?(x=w20, y=w641) -> (0:w430:bool)
    "Boolean 5" <- w430
    n160 = Greater?(x=w625, y=0.0) -> (0:w617:bool)
    n161 = Greater?(x=w70, y=w69) -> (0:w74:bool)
    n162 = Less?(x=w122, y=w123) -> (x < y?=→"Boolean 75":bool)
    n163 = Less?(x=w118, y=w119) -> (x < y?=→"Boolean 89":bool)
    n164 = Greater?(x=w612, y=0.0) -> (0:w608:bool)
    n165 = Less?(x=w126, y=w127) -> (x < y?=→"Boolean 45":bool)
    n166 = Less?(x=w132, y=w130) -> (x < y?=→"Boolean 18":bool)
    n167 = Or(x=w80, y=w79) -> (x .or. y?=→"Boolean 67":bool)
    n168 = Less?(x=w91, y=4.0) -> (x < y?=w94:bool)
    n169 = Less?(x=w105, y=2.8) -> (x < y?=w101:bool)
    n170 = Greater?(x=w105, y=w104) -> (0:w103:bool)
    n171 = Less?(x=w64, y=2.85) -> (x < y?=w59:bool)
    n172 = Less?(x=w110, y=5.0) -> (x < y?=w107:bool)
    n173 = Less?(x=w70, y=w73) -> (x < y?=w72:bool)
    n174 = And(x=w72, y=w74) -> (x .and. y?=→"Boolean 30":bool)
    n175 = Greater?(x=w64, y=2.0) -> (0:w57:bool)
    n176 = Or(x=w560, y=w559) -> (x .or. y?=w450:bool)
    "Boolean 43" <- w450
    n177 = Or(x=w295, y=w294) -> (x .or. y?=w272:bool)
    "Boolean 85" <- w272
    n178 = Or(x=w286, y=w285) -> (x .or. y?=w269:bool)
    "Boolean 87" <- w269
    n179 = Or(x=w569, y=w568) -> (x .or. y?=w448:bool)
    "Boolean 41" <- w448
    n180 = Or(x=w554, y=w553) -> (x .or. y?=w452:bool)
    "Boolean 47" <- w452
    n181 = Or(x=w548, y=w547) -> (x .or. y?=w454:bool)
    "Boolean 49" <- w454
    n182 = Or(x=w335, y=w334) -> (x .or. y?=w309:bool)
    "Boolean 79" <- w309
    n183 = Or(x=w326, y=w325) -> (x .or. y?=w308:bool)
    "Boolean 81" <- w308
    n184 = Or(x=w542, y=w541) -> (x .or. y?=w456:bool)
    "Boolean 51" <- w456
    n185 = Or(x=w536, y=w535) -> (x .or. y?=w457:bool)
    "Boolean 53" <- w457
    n186 = Or(x=w528, y=w527) -> (x .or. y?=w461:bool)
    "Boolean 55" <- w461
    n187 = Or(x=w522, y=w521) -> (x .or. y?=w463:bool)
    "Boolean 57" <- w463
    n188 = Or(x=w516, y=w515) -> (x .or. y?=w505:bool)
    "Boolean 59" <- w505
    n189 = Or(x=w344, y=w343) -> (x .or. y?=w312:bool)
    "Boolean 77" <- w312
    n190 = Or(x=w304, y=w303) -> (x .or. y?=w273:bool)
    "Boolean 83" <- w273
    n191 = Or(x=w425, y=w424) -> (x .or. y?=w366:bool)
    "Boolean 61" <- w366
    n192 = Or(x=w353, y=w352) -> (x .or. y?=w314:bool)
    "Boolean 73" <- w314
    n193 = Or(x=w416, y=w415) -> (x .or. y?=w365:bool)
    "Boolean 63" <- w365
    n194 = Or(x=w407, y=w406) -> (x .or. y?=w363:bool)
    "Boolean 65" <- w363
    n195 = Or(x=w398, y=w397) -> (x .or. y?=w360:bool)
    n196 = Or(x=w390, y=w389) -> (x .or. y?=w356:bool)
    "Boolean 69" <- w356
    n197 = Or(x=w381, y=w380) -> (x .or. y?=w359:bool)
    "Boolean 71" <- w359
    n198 = Less?(x=w48, y=2.75) -> (x < y?=w50:bool)
    n199 = Greater?(x=w110, y=w109) -> (0:w108:bool)
    n200 = Greater?(x=w112, y=13.2) -> (0:w601:bool)
    n201 = Or(x=w601, y=w600) -> (x .or. y?=w63:bool)
    "Boolean 16" <- w63
    n202 = Greater?(x=w48, y=2.0) -> (0:w51:bool)
    n203 = Less?(x=w37, y=2.75) -> (x < y?=w42:bool)
    n204 = Greater?(x=w37, y=2.0) -> (0:w43:bool)
    n205 = And(x=w103, y=w101) -> (x .and. y?=w102:bool)
    "Boolean 24" <- w102
    n206 = And(x=w59, y=w57) -> (x .and. y?=→"Boolean 33":bool)
    n207 = And(x=w108, y=w107) -> (x .and. y?=→"Boolean 21":bool)
    n208 = And(x=w50, y=w51) -> (x .and. y?=→"Boolean 36":bool)
    n209 = Greater?(x=w91, y=6.0) -> (0:w95:bool)
    n210 = And(x=w42, y=w43) -> (x .and. y?=→"Boolean 39":bool)
    n211 = Greater?(x=w122, y=w123) -> (0:→"Boolean 46":bool)
    n212 = Greater?(x=w118, y=w119) -> (0:→"Boolean 76":bool)
    n213 = Greater?(x=w126, y=w127) -> (0:→"Boolean 19":bool)
    n214 = Greater?(x=w132, y=w130) -> (0:→"Boolean 9":bool)
    n215 = Greater?(x=w77, y=w81) -> (0:w82:bool)
    n216 = Less?(x=w77, y=w76) -> (x < y?=w83:bool)
    n217 = Less?(x=w134, y=w639) -> (x < y?=w432:bool)
    "Boolean 7" <- w432
    n218 = Greater?(x=w139, y=25.0) -> (0:w135:bool)
    n219 = Less?(x=w139, y=27.0) -> (x < y?=w136:bool)
    n220 = Less?(x=w70, y=10.0) -> (x < y?=w588:bool)
    n221 = Or(x=w591, y=w588) -> (x .or. y?=w587:bool)
    "Boolean 29" <- w587
    n222 = Or(x=w95, y=w94) -> (x .or. y?=w96:bool)
    "Boolean 26" <- w96
    n223 = Less?(x=w114, y=27.0) -> (x < y?=w117:bool)
    n224 = Greater?(x=w70, y=10.0) -> (0:w66:bool)
    n225 = Not(x=w450) -> (.not. x?=→"Boolean 44":bool)
    n226 = Not(x=w272) -> (.not. x?=→"Boolean 86":bool)
    n227 = Not(x=w269) -> (.not. x?=→"Boolean 88":bool)
    n228 = Greater?(x=w114, y=25.0) -> (0:w113:bool)
    n229 = Not(x=w448) -> (.not. x?=→"Boolean 42":bool)
    n230 = Not(x=w452) -> (.not. x?=→"Boolean 48":bool)
    n231 = Not(x=w454) -> (.not. x?=→"Boolean 50":bool)
    n232 = Not(x=w309) -> (.not. x?=→"Boolean 80":bool)
    n233 = Not(x=w308) -> (.not. x?=→"Boolean 82":bool)
    n234 = Not(x=w456) -> (.not. x?=→"Boolean 52":bool)
    n235 = Not(x=w457) -> (.not. x?=→"Boolean 54":bool)
    n236 = Not(x=w461) -> (.not. x?=→"Boolean 56":bool)
    n237 = Not(x=w463) -> (.not. x?=→"Boolean 58":bool)
    n238 = Not(x=w505) -> (.not. x?=→"Boolean 60":bool)
    n239 = Not(x=w312) -> (.not. x?=→"Boolean 78":bool)
    n240 = Not(x=w273) -> (.not. x?=→"Boolean 84":bool)
    n241 = Not(x=w366) -> (.not. x?=→"Boolean 62":bool)
    n242 = Not(x=w314) -> (.not. x?=→"Boolean 74":bool)
    n243 = Not(x=w365) -> (.not. x?=→"Boolean 64":bool)
    n244 = Not(x=w363) -> (.not. x?=→"Boolean 66":bool)
    n245 = Not(x=w356) -> (.not. x?=→"Boolean 70":bool)
    n246 = Not(x=w359) -> (.not. x?=→"Boolean 72":bool)
    n247 = And(x=w83, y=w82) -> (x .and. y?=→"Boolean 68":bool)
    n248 = Less?(x=w70, y=w69) -> (x < y?=w67:bool)
    n249 = Less?(x=w23, y=w22) -> (x < y?=w31:bool)
    n250 = And(x=w136, y=w135) -> (x .and. y?=w137:bool)
    "Boolean 11" <- w137
    n251 = Greater?(x=w110, y=5.0) -> (0:w34:bool)
    n252 = Less?(x=w30, y=w29) -> (x < y?=w35:bool)
    n253 = Greater?(x=w105, y=2.8) -> (0:w32:bool)
    n254 = Less?(x=w64, y=2.0) -> (x < y?=→"Boolean 34":bool)
    n255 = And(x=w67, y=w66) -> (x .and. y?=→"Boolean 31":bool)
    n256 = And(x=w117, y=w113) -> (x .and. y?=w116:bool)
    "Boolean 14" <- w116
    n257 = Not(x=w63) -> (.not. x?=→"Boolean 17":bool)
    n258 = Or(x=w32, y=w31) -> (x .or. y?=→"Boolean 25":bool)
    n259 = Or(x=w34, y=w35) -> (x .or. y?=→"Boolean 22":bool)
    n260 = Less?(x=w37, y=2.0) -> (x < y?=→"Boolean 40":bool)
    n261 = Less?(x=w48, y=2.0) -> (x < y?=→"Boolean 37":bool)
    n262 = Equal?(x=w432, y=w431) -> (x = y?=w467:bool)
    n263 = Equal?(x=w430, y=w429) -> (x = y?=w464:bool)
    n264 = Equal?(x=w448, y=w183) -> (x = y?=w482:bool)
    n265 = Equal?(x=w450, y=w449) -> (x = y?=w485:bool)
    n266 = Equal?(x=w272, y=w271) -> (x = y?=w289:bool)
    n267 = Equal?(x=w269, y=w270) -> (x = y?=w280:bool)
    n268 = Equal?(x=w452, y=w451) -> (x = y?=w488:bool)
    n269 = Equal?(x=w457, y=w458) -> (x = y?=w497:bool)
    n270 = Equal?(x=w309, y=w310) -> (x = y?=w329:bool)
    n271 = Equal?(x=w308, y=w307) -> (x = y?=w320:bool)
    n272 = Equal?(x=w461, y=w460) -> (x = y?=w499:bool)
    n273 = Equal?(x=w463, y=w462) -> (x = y?=w502:bool)
    n274 = Equal?(x=w505, y=w506) -> (x = y?=w507:bool)
    n275 = Equal?(x=w312, y=w311) -> (x = y?=w338:bool)
    n276 = Equal?(x=w273, y=w274) -> (x = y?=w298:bool)
    n277 = Equal?(x=w454, y=w453) -> (x = y?=w491:bool)
    n278 = Equal?(x=w366, y=w367) -> (x = y?=w419:bool)
    n279 = Equal?(x=w314, y=w313) -> (x = y?=w347:bool)
    n280 = Or(x=w587, y=w74) -> (x .or. y?=w447:bool)
    n281 = Equal?(x=w456, y=w455) -> (x = y?=w494:bool)
    n282 = Equal?(x=w365, y=w364) -> (x = y?=w410:bool)
    n283 = Equal?(x=w363, y=w362) -> (x = y?=w401:bool)
    n284 = Equal?(x=w360, y=w361) -> (x = y?=w393:bool)
    n285 = Equal?(x=w356, y=w357) -> (x = y?=w384:bool)
    n286 = Equal?(x=w359, y=w358) -> (x = y?=w375:bool)
    n287 = Not(x=w96) -> (.not. x?=→"Boolean 27":bool)
    n288 = Not(x=w467) -> (.not. x?=w468:bool)
    n289 = Not(x=w464) -> (.not. x?=w465:bool)
    n290 = Not(x=w482) -> (.not. x?=w483:bool)
    n291 = xnode "Steinhart-Hart"("X1"="A", "X2"="B", "X3"="C") -> ("Result"=w634:dbl)  [unwired: 2 in, 1 out]
    n292 = Less?(x=w139, y=25.0) -> (x < y?=w616:bool)
    n293 = And(x=w617, y=w616) -> (x .and. y?=w613:bool)
    "Boolean 10" <- w613
    n294 = Not(x=w485) -> (.not. x?=w486:bool)
    n295 = Not(x=w289) -> (.not. x?=w290:bool)
    n296 = Not(x=w280) -> (.not. x?=w281:bool)
    n297 = Less?(x=w114, y=25.0) -> (x < y?=w607:bool)
    n298 = And(x=w608, y=w607) -> (x .and. y?=w604:bool)
    "Boolean 13" <- w604
    n299 = Not(x=w488) -> (.not. x?=w489:bool)
    n300 = Not(x=w497) -> (.not. x?=w498:bool)
    n301 = Not(x=w329) -> (.not. x?=w330:bool)
    n302 = Not(x=w320) -> (.not. x?=w321:bool)
    n303 = Not(x=w499) -> (.not. x?=w500:bool)
    n304 = Not(x=w502) -> (.not. x?=w503:bool)
    n305 = Not(x=w507) -> (.not. x?=w508:bool)
    n306 = Not(x=w338) -> (.not. x?=w339:bool)
    n307 = Not(x=w298) -> (.not. x?=w299:bool)
    n308 = Not(x=w491) -> (.not. x?=w492:bool)
    n309 = Not(x=w419) -> (.not. x?=w420:bool)
    n310 = Not(x=w347) -> (.not. x?=w348:bool)
    n311 = Not(x=w494) -> (.not. x?=w495:bool)
    n312 = Not(x=w410) -> (.not. x?=w411:bool)
    n313 = Not(x=w401) -> (.not. x?=w402:bool)
    n314 = Not(x=w393) -> (.not. x?=w394:bool)
    n315 = Not(x=w384) -> (.not. x?=w385:bool)
    n316 = Not(x=w375) -> (.not. x?=w376:bool)
    n317 = Greater?(x=w77, y=w75) -> (0:w86:bool)
    n318 = Less?(x=w77, y=w81) -> (x < y?=w87:bool)
    n319 = And(x=w432, y=w468) -> (x .and. y?=w469:bool)
    n320 = case shown="True" w469 {
      frame False {
      }
      frame True {
        n321 = call <vilib>:"Beep.vi"() -> ()  [unwired: 12 in]
      }
    }
    n322 = And(x=w430, y=w465) -> (x .and. y?=w466:bool)
    n323 = case shown="True" w466 {
      frame False {
      }
      frame True {
        n324 = call <vilib>:"Beep.vi"() -> ()  [unwired: 12 in]
      }
    }
    n325 = Or(x=w28, y=w107) -> (x .or. y?=w443:bool)
    n326 = And(x=w448, y=w483) -> (x .and. y?=w484:bool)
    n327 = case shown="True" w484 {
      frame False {
      }
      frame True {
        n328 = call <vilib>:"Beep.vi"() -> ()  [unwired: 12 in]
      }
    }
    n329 = And(x=w450, y=w486) -> (x .and. y?=w487:bool)
    n330 = case shown="True" w487 {
      frame False {
      }
      frame True {
        n331 = call <vilib>:"Beep.vi"() -> ()  [unwired: 12 in]
      }
    }
    n332 = And(x=w272, y=w290) -> (x .and. y?=w291:bool)
    n333 = case shown="True" w291 {
      frame False {
      }
      frame True {
        n334 = call <vilib>:"Beep.vi"() -> ()  [unwired: 12 in]
      }
    }
    n335 = And(x=w269, y=w281) -> (x .and. y?=w282:bool)
    n336 = case shown="True" w282 {
      frame False {
      }
      frame True {
        n337 = call <vilib>:"Beep.vi"() -> ()  [unwired: 12 in]
      }
    }
    n338 = And(x=w452, y=w489) -> (x .and. y?=w490:bool)
    n339 = case shown="True" w490 {
      frame False {
      }
      frame True {
        n340 = call <vilib>:"Beep.vi"() -> ()  [unwired: 12 in]
      }
    }
    n341 = And(x=w457, y=w498) -> (x .and. y?=w459:bool)
    n342 = case shown="True" w459 {
      frame False {
      }
      frame True {
        n343 = call <vilib>:"Beep.vi"() -> ()  [unwired: 12 in]
      }
    }
    n344 = And(x=w309, y=w330) -> (x .and. y?=w331:bool)
    n345 = case shown="True" w331 {
      frame False {
      }
      frame True {
        n346 = call <vilib>:"Beep.vi"() -> ()  [unwired: 12 in]
      }
    }
    n347 = And(x=w308, y=w321) -> (x .and. y?=w322:bool)
    n348 = case shown="True" w322 {
      frame False {
      }
      frame True {
        n349 = call <vilib>:"Beep.vi"() -> ()  [unwired: 12 in]
      }
    }
    n350 = And(x=w461, y=w500) -> (x .and. y?=w501:bool)
    n351 = case shown="True" w501 {
      frame False {
      }
      frame True {
        n352 = call <vilib>:"Beep.vi"() -> ()  [unwired: 12 in]
      }
    }
    n353 = And(x=w463, y=w503) -> (x .and. y?=w504:bool)
    n354 = case shown="True" w504 {
      frame False {
      }
      frame True {
        n355 = call <vilib>:"Beep.vi"() -> ()  [unwired: 12 in]
      }
    }
    n356 = And(x=w505, y=w508) -> (x .and. y?=w509:bool)
    n357 = case shown="True" w509 {
      frame False {
      }
      frame True {
        n358 = call <vilib>:"Beep.vi"() -> ()  [unwired: 12 in]
      }
    }
    n359 = And(x=w312, y=w339) -> (x .and. y?=w340:bool)
    n360 = case shown="True" w340 {
      frame False {
      }
      frame True {
        n361 = call <vilib>:"Beep.vi"() -> ()  [unwired: 12 in]
      }
    }
    n362 = And(x=w273, y=w299) -> (x .and. y?=w300:bool)
    n363 = case shown="True" w300 {
      frame False {
      }
      frame True {
        n364 = call <vilib>:"Beep.vi"() -> ()  [unwired: 12 in]
      }
    }
    n365 = And(x=w454, y=w492) -> (x .and. y?=w493:bool)
    n366 = case shown="True" w493 {
      frame False {
      }
      frame True {
        n367 = call <vilib>:"Beep.vi"() -> ()  [unwired: 12 in]
      }
    }
    n368 = And(x=w366, y=w420) -> (x .and. y?=w421:bool)
    n369 = case shown="True" w421 {
      frame False {
      }
      frame True {
        n370 = call <vilib>:"Beep.vi"() -> ()  [unwired: 12 in]
      }
    }
    n371 = And(x=w314, y=w348) -> (x .and. y?=w349:bool)
    n372 = case shown="True" w349 {
      frame False {
      }
      frame True {
        n373 = call <vilib>:"Beep.vi"() -> ()  [unwired: 12 in]
      }
    }
    n374 = And(x=w456, y=w495) -> (x .and. y?=w496:bool)
    n375 = case shown="True" w496 {
      frame False {
      }
      frame True {
        n376 = call <vilib>:"Beep.vi"() -> ()  [unwired: 12 in]
      }
    }
    n377 = And(x=w365, y=w411) -> (x .and. y?=w412:bool)
    n378 = case shown="True" w412 {
      frame False {
      }
      frame True {
        n379 = call <vilib>:"Beep.vi"() -> ()  [unwired: 12 in]
      }
    }
    n380 = And(x=w363, y=w402) -> (x .and. y?=w403:bool)
    n381 = case shown="True" w403 {
      frame False {
      }
      frame True {
        n382 = call <vilib>:"Beep.vi"() -> ()  [unwired: 12 in]
      }
    }
    n383 = And(x=w360, y=w394) -> (x .and. y?=w395:bool)
    n384 = case shown="True" w395 {
      frame False {
      }
      frame True {
        n385 = call <vilib>:"Beep.vi"() -> ()  [unwired: 12 in]
      }
    }
    n386 = And(x=w356, y=w385) -> (x .and. y?=w386:bool)
    n387 = case shown="True" w386 {
      frame False {
      }
      frame True {
        n388 = call <vilib>:"Beep.vi"() -> ()  [unwired: 12 in]
      }
    }
    n389 = And(x=w359, y=w376) -> (x .and. y?=w377:bool)
    n390 = case shown="True" w377 {
      frame False {
      }
      frame True {
        n391 = call <vilib>:"Beep.vi"() -> ()  [unwired: 12 in]
      }
    }
    n392 = And(x=w87, y=w86) -> (x .and. y?=→"Boolean 90":bool)
    n393 = Or(x=w25, y=w102) -> (x .or. y?=w445:bool)
    n394 = Greater?(x=w139, y=27.0) -> (0:→"Boolean 12":bool)
    n395 = Greater?(x=w114, y=27.0) -> (0:→"Boolean 15":bool)
    n396 = call "Convert from Dynamic Data"("Dynamic Data Type"=w634) -> ("Array"=w633:dbl[])  [unwired: 3 in]
    n397 = Or(x=w613, y=w137) -> (x .or. y?=w89:bool)
    n398 = Or(x=w604, y=w116) -> (x .or. y?=w434:bool)
    n399 = Build Array(w134, w126) -> (w626:dbl[])
    n400 = Build Array(w64, w48, w37) -> (w579:dbl[])
    n401 = Build Array(w20, w122) -> (w621:dbl[])
    n402 = Build Array(w132, w118) -> (w619:dbl[])
    n403 = Build Array(w531, w19, w18) -> (w144:dbl[])
    n404 = Build Array (concatenate)(w636, w633) -> (w635:dbl[][])
    n405 = Build Array (concatenate)(w597, w110) -> (w4:dbl[])
    "Iout" <- w4
    n406 = Build Array (concatenate)(w593, w105) -> (w5:dbl[])
    "I12d+" <- w5
    n407 = Build Array(w565, w15, w14) -> (w564:dbl[])
    n408 = Build Array (concatenate)(w637, w626) -> (w1:dbl[][])
    "+1 Order TECs" <- w1
    n409 = Build Array (concatenate)(w620, w621) -> (w2:dbl[][])
    "-1 Order TECs" <- w2
    n410 = Build Array (concatenate)(w618, w619) -> (w3:dbl[][])
    "0 Order TECs" <- w3
    n411 = Build Array(w319, w153, w318, w317) -> (w315:dbl[])
    n412 = Equal?(x=w447, y=w446) -> (x = y?=w479:bool)
    n413 = Equal?(x=w443, y=w442) -> (x = y?=w473:bool)
    n414 = Equal?(x=w445, y=w444) -> (x = y?=w476:bool)
    n415 = Build Array(w510, w17, w16) -> (w512:dbl[])
    n416 = Build Array(w374, w373, w372, w371, w370) -> (w369:dbl[])
    n417 = Build Array(w279, w278, w277) -> (w276:dbl[])
    n418 = Not(x=w479) -> (.not. x?=w480:bool)
    n419 = Not(x=w473) -> (.not. x?=w474:bool)
    n420 = Not(x=w476) -> (.not. x?=w477:bool)
    n421 = Build Array (concatenate)(w182, w70) -> (w6:dbl[])
    "I5s" <- w6
    n422 = Build Array (concatenate)(w580, w579) -> (w7:dbl[][])
    "TEC Currents" <- w7
    n423 = Build Array (concatenate)(w275, w276) -> (w13:dbl[][])
    "PCU" <- w13
    n424 = Build Array (concatenate)(w563, w564) -> (w8:dbl[][])
    "Reservoir" <- w8
    n425 = Build Array (concatenate)(w532, w144) -> (w9:dbl[][])
    "Cold Fingers" <- w9
    n426 = And(x=w447, y=w480) -> (x .and. y?=w481:bool)
    n427 = case shown="True" w481 {
      frame False {
      }
      frame True {
        n428 = call <vilib>:"Beep.vi"() -> ()  [unwired: 12 in]
      }
    }
    n429 = Equal?(x=w63, y=w176) -> (x = y?=w470:bool)
    n430 = And(x=w443, y=w474) -> (x .and. y?=w475:bool)
    n431 = case shown="True" w475 {
      frame False {
      }
      frame True {
        n432 = call <vilib>:"Beep.vi"() -> ()  [unwired: 12 in]
      }
    }
    n433 = Build Array (concatenate)(w511, w512) -> (w10:dbl[][])
    "Back Plates" <- w10
    n434 = And(x=w445, y=w477) -> (x .and. y?=w478:bool)
    n435 = case shown="True" w478 {
      frame False {
      }
      frame True {
        n436 = call <vilib>:"Beep.vi"() -> ()  [unwired: 12 in]
      }
    }
    n437 = Build Array (concatenate)(w316, w315) -> (w12:dbl[][])
    "CONT" <- w12
    n438 = Build Array (concatenate)(w368, w369) -> (w11:dbl[][])
    "COMP" <- w11
    n439 = Not(x=w470) -> (.not. x?=w471:bool)
    n440 = Equal?(x=w89, y=w435) -> (x = y?=w436:bool)
    n441 = Equal?(x=w434, y=w433) -> (x = y?=w439:bool)
    n442 = And(x=w63, y=w471) -> (x .and. y?=w472:bool)
    n443 = case shown="True" w472 {
      frame False {
      }
      frame True {
        n444 = call <vilib>:"Beep.vi"() -> ()  [unwired: 12 in]
      }
    }
    n445 = Not(x=w436) -> (.not. x?=w437:bool)
    n446 = Not(x=w439) -> (.not. x?=w440:bool)
    n447 = And(x=w89, y=w437) -> (x .and. y?=w438:bool)
    n448 = case shown="True" w438 {
      frame False {
      }
      frame True {
        n449 = call <vilib>:"Beep.vi"() -> ()  [unwired: 12 in]
      }
    }
    n450 = And(x=w434, y=w440) -> (x .and. y?=w441:bool)
    n451 = case shown="True" w441 {
      frame False {
      }
      frame True {
        n452 = call <vilib>:"Beep.vi"() -> ()  [unwired: 12 in]
      }
    }
  }
  n453 = invoke on="Power" class="SubPanel" method="Remove VI"() -> ()  [unwired: 3 in, 3 out]
  n454 = while {
    stop <- w1570 stop-if-true
    n455 = local read "stop 2"() -> (w1570:bool)
    n456 = control-ref of="Output Array"() -> (w1569:refnum<vi>)
    n457 = case shown="True" "?" {
      tunnel: w1569 -> [_ w1585]
      frame False {
      }
      frame True {
        n458 = call "MOSES Background 4.vi"("Array Input"=w1585) -> ("PSU"=→"PSU":dbl[], "Values to Output"=w1584:T5, "Power Supply Filter Input"=→"Power Supply Filter Input":dbl[], "ROE"=→"ROE":dbl[])  [unwired: 1 in]
        n459 = Unbundle By Name(w1584) -> ("T5V, Thermal 5V power voltage"=→"Thermal 5V power":dbl, "S28V, Shutter 28V power voltage"=→"Shutter 28V power":dbl, "HAFV, H-alpha filter voltage"=→"H-alpha filter":dbl, "HACV, H-alpha camera voltage"=→"H-alpha camera":dbl, "Ipf12+, Premod filter positive 12V input current"=→"Premod filter positive 12V input":dbl, "I_pf5, Premod filter 5V input current"=→"Premod filter 5V input":dbl, "S28I, Shutter 28V power current"=→"Shutter 28V power":dbl, "HAFI, H-alpha filter current"=→"H-alpha filter":dbl, "ROE_PSV, ROE power supply input voltage"=→"ROE power supply input":dbl, "ROE_PSI, ROE power supply input current"=→"ROE power supply input":dbl)  [unwired: 9 out]
      }
    }
  }
